vi "SVM Dense Train NU_SVR.vi"(7 "Options":T6={"cache_size"=200.0, "eps"=0.001, "shrinking"=TRUE, "probability"=FALSE}, 8 "error in (no error)":errorcluster, 9 "Param NU_SVR":T7={"C"=1.0, "nu"=0.5}, 10 "Kernel":T8, 11 "Dense problem":T5) -> (0 "error out":errorcluster, 3 "Model":T1)   [LabVIEW 2015]
doc: "This function constructs and returns an SVM model according to the given training data and parameters."
uses:
  LibSVM Sparse/Controls/Kernel.ctl
  LibSVM Sparse/Wrapper API/Controls/svm_kernel_type.ctl
  LibSVM Sparse/Controls/Parameters NU_SVR.ctl
  LibSVM Sparse/Controls/Options Training.ctl
  Wrapper API/Controls/svmdense_problem.ctl
  Wrapper API/Controls/svmdense_model.ctl
  LibSVM Sparse/Wrapper API/Controls/svm_parameter.ctl
  LibSVM Sparse/Wrapper API/Controls/svm_type.ctl
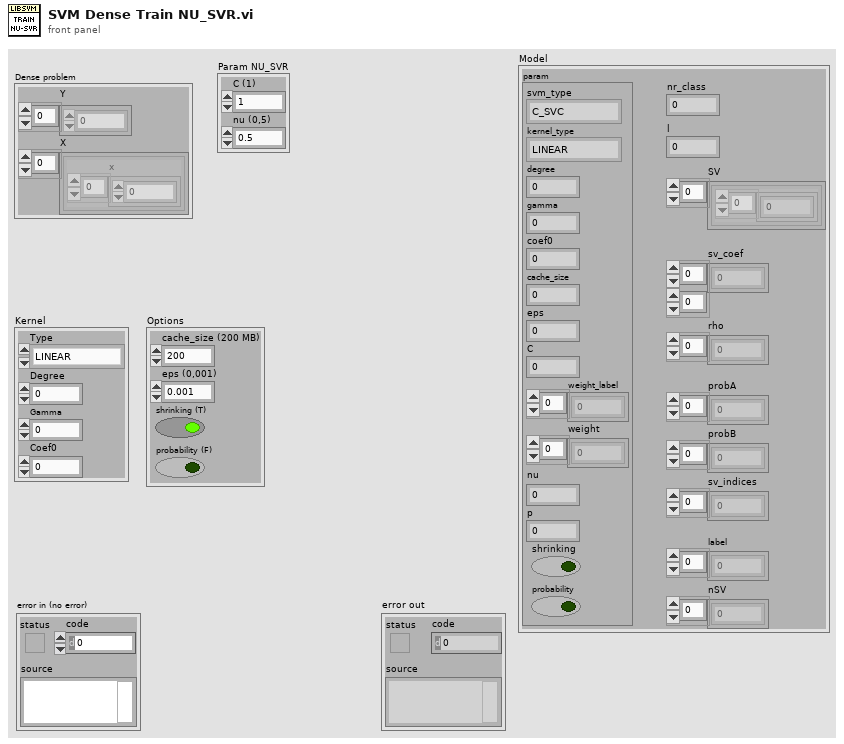
[diagram p1: front panel]
types:
  T1 = typedef "svmdense_model.ctl" = cluster{"param":T2, "nr_class":i32, "l":i32, "SV":cluster{"Array":dbl[]}[], "sv_coef":dbl[][], "rho":dbl[], "probA":dbl[], "probB":dbl[], "sv_indices":i32[], "label":i32[], "nSV":i32[]}
  T2 = typedef "svm_parameter.ctl" = cluster{"svm_type":T3, "kernel_type":T4, "degree":i32, "gamma":dbl, "coef0":dbl, "cache_size":dbl, "eps":dbl, "C":dbl, "weight_label":i32[], "weight":dbl[], "nu":dbl, "p":dbl, "shrinking":bool, "probability":bool}
  T3 = typedef "svm_type.ctl" = enum32{"C_SVC", "NU_SVC", "ONE_CLASS", "EPSILON_SVR", "NU_SVR"}
  T4 = typedef "svm_kernel_type.ctl" = enum32{"LINEAR", "POLY", "RBF", "SIGMOID", "PRECOMPUTED"}
  T5 = typedef "svmdense_problem.ctl" = cluster{"Y":dbl[], "X":cluster{"x":dbl[]}[]}
  T6 = typedef "Options Training.ctl" = cluster{"cache_size":dbl, "eps":dbl, "shrinking":bool, "probability":bool}
  T7 = typedef "Parameters NU_SVR.ctl" = cluster{"C":dbl, "nu":dbl}
  T8 = typedef "Kernel.ctl" = cluster{"Type":T4, "Degree":i32, "Gamma":dbl, "Coef0":dbl}
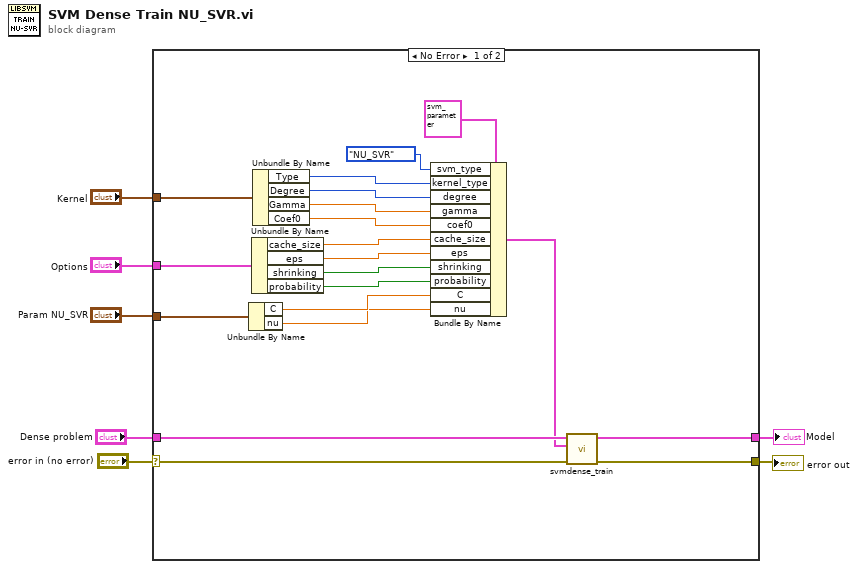
[diagram p0: block diagram]
diagram:
  n1 = case shown="No Error" "error in (no error)" {
    selector: "error in (no error)" -> [w10 w28]
    tunnel: [w8 w28] -> w7
    tunnel: "Dense problem" -> [w12 _]
    tunnel: "Kernel" -> [w26 _]
    tunnel: [w9 _] -> w1
    tunnel: "Options" -> [w17 _]
    tunnel: "Param NU_SVR" -> [w18 _]
    frame No Error {
      n2 = Unbundle By Name(w18) -> ("C"=w14:dbl, "nu"=w13:dbl)
      n3 = Unbundle By Name(w17) -> ("cache_size"=w20:dbl, "eps"=w19:dbl, "shrinking"=w16:bool, "probability"=w15:bool)
      n4 = Unbundle By Name(w26) -> ("Type"=w25:T4, "Degree"=w24:i32, "Gamma"=w23:dbl, "Coef0"=w22:dbl)
      n5 = Bundle By Name(cluster=T2 {"svm_type"=enum."C_SVC", "kernel_type"=enum."LINEAR", "degree"=0, "gamma"=0.0, "coef0"=0.0, "cache_size"=0.0, "eps"=0.0, "C"=0.0, "weight_label"=[], "weight"=[], "nu"=0.0, "p"=0.0, "shrinking"=FALSE, "probability"=FALSE} ("svm_parameter"), "svm_type"=svm_type."NU_SVR", "kernel_type"=w25, "degree"=w24, "gamma"=w23, "coef0"=w22, "cache_size"=w20, "eps"=w19, "shrinking"=w16, "probability"=w15, "C"=w14, "nu"=w13) -> (w11:T2)
      n6 = call "svmdense_train.vi"("error in (no error)"=w10, "Parameters"=w11, "Problem"=w12) -> ("error out"=w8:errorcluster, "Model"=w9:T1)  [unwired: 7 in]
    }
    frame Error {
    }
  }
  "error out" <- w7
  "Model" <- w1
